vi "Z Aux Set Ip.vi"(8 "error in (no error)":errorcluster caption="错误输入（无错误）", 10 "ipaddress":string, 11 "handle":u32) -> (0 "error out":errorcluster caption="错误输出", 1 "function return":i32, 2 "ipaddress out":string, 3 "handle out":u32)   [LabVIEW 2015, in "zauxdll.lvlib"]
doc: "int32 __stdcall ZAux_SetIp(ZMC_HANDLE handle, char * ipaddress);"
uses:
  zauxdll.lvlib
  Radar - 2015 32bit_autoqueue_angle_0319/zauxdll-2014/zauxdll.dll
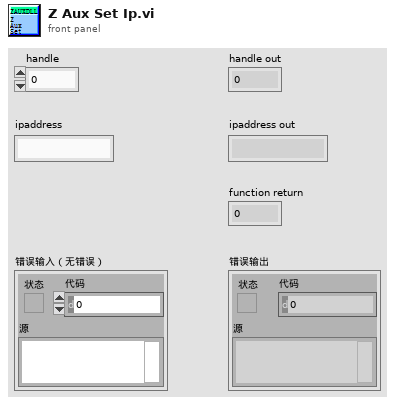
[diagram p1: front panel]
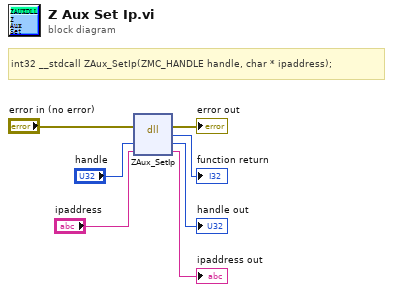
[diagram p0: block diagram]
diagram:
  # "int32 __stdcall ZAux_SetIp(ZMC_HANDLE handle, char * ipaddress);"
  n1 = dll-call lib="D:/vicomm case/cub/0717/Radar - 2015 32bit_autoqueue_angle_0319/zauxdll-2014/zauxdll.*" fn="ZAux_SetIp"(error in="error in (no error)", "handle"="handle", "ipaddress"="ipaddress") -> (error out=→"error out":errorcluster, →"function return":i32, "handle"=→"handle out":u32, "ipaddress"=→"ipaddress out":string)  [unwired: 2 in, 1 out]
